vi "Untitled 2.vi"   [LabVIEW 2021]
uses:
  Classes/Workspace/Component/Component Tray.lvclass
  Classes/Controller/Controller.lvclass
types:
  T1 = typedef "Controller.lvclass/Controllers.ctl" = cluster{"I-O.lvclass":refnum<class "I-O.lvclass">, "Gantry":refnum<k24>, "Dispenser":refnum<visa-resource-name>}
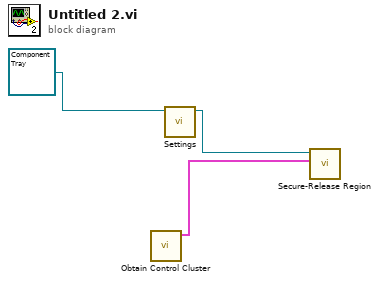
[diagram p0: block diagram]
diagram:
  n1 = call "Obtain Control Cluster.vi"() -> ("Control Out"=w1:T1)  [unwired: 11 in]
  n2 = call-dynamic "Settings.vi"("Component in"=refnum<class "Component Tray.lvclass"> refnum ("Component Tray.lvclass")) -> ("Component out"=w2:refnum<class "Component Tray.lvclass">)  [unwired: 9 in, 1 out]
  n3 = call-dynamic "Secure-Release Region.vi"("Control In"=w1, "Workspace in"=w2) -> ()  [unwired: 7 in, 3 out]
